vi "avgCoherence.vi"(3 "error in (no error)":errorcluster, 4 "frequency (cycles/period)":dbl, 5 "x2":dbl[](array[numeric]), 6 "x1":dbl[](array[numeric])) -> (0 "error out":errorcluster, 1 "coherence":dbl[](array[numeric]), 2 "coherence at frequency":dbl)   [LabVIEW 2017]
uses:
  <vilib>/measure/maspectr.llb/Frequency Response Function (Mag-Phase) 1-1.vi
  <vilib>/measure/NI_MAPro.lvlib
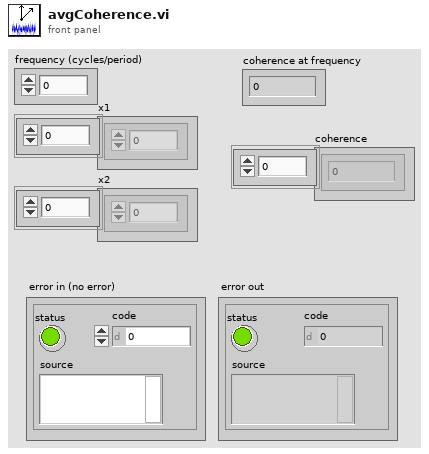
[diagram p1: front panel]
types:
  T1 = cluster{"averaging mode":enum16{"No averaging", "Vector averaging", "RMS averaging", "Peak hold"}, "weighting mode":enum16{"Linear", "Exponential"}, "number of averages":u32}
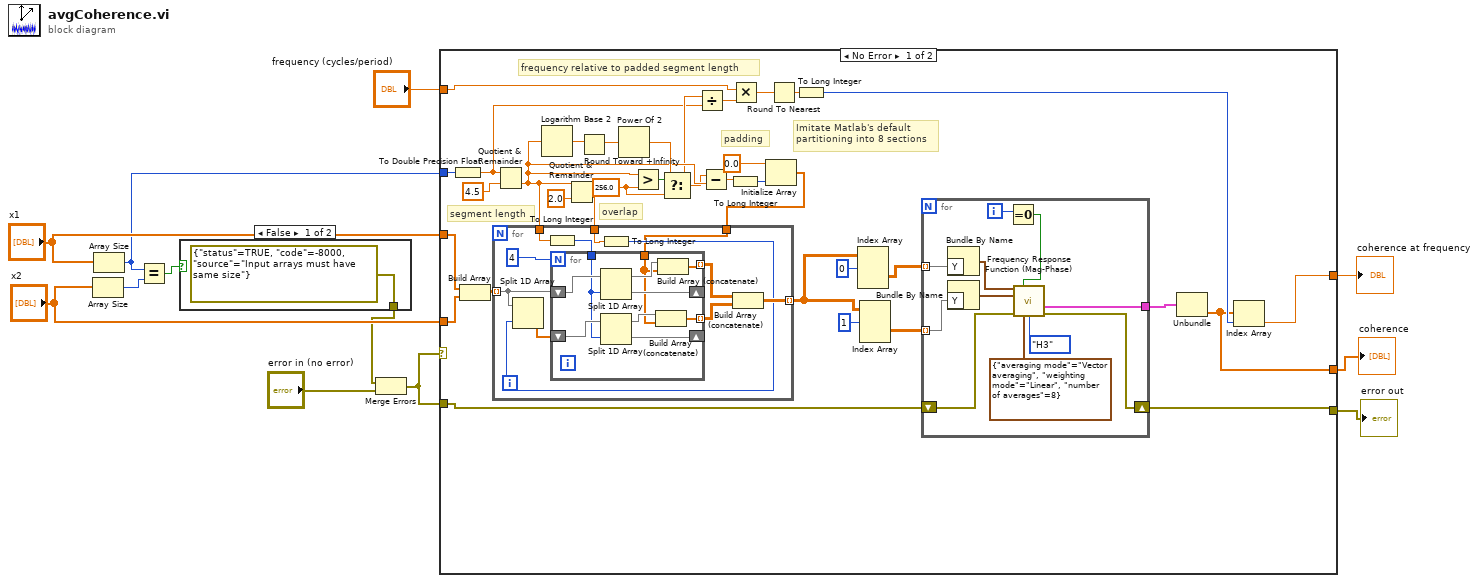
[diagram p0: block diagram]
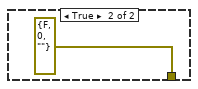
[diagram p2: hidden frame]
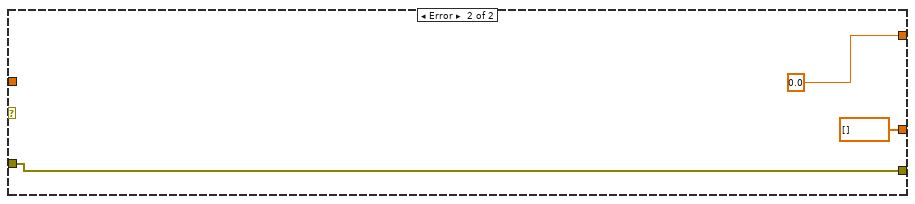
[diagram p3: hidden frame]
diagram:
  n1 = Array Size(array="x2") -> (size(s)=w10:i32)
  n2 = Array Size(array="x1") -> (size(s)=w5:i32)
  n3 = Equal?(x=w5, y=w10) -> (x = y?=w9:bool)
  n4 = case shown="False" w9 {
    tunnel: [errorcluster {"status"=TRUE, "code"=-8000, "source"="Input arrays must have same size"} ("error constant") errorcluster {"status"=FALSE, "code"=0, "source"=""} ("error constant")] -> w8
    frame False {
    }
    frame True {
    }
  }
  n5 = Merge Errors(w8, "error in (no error)") -> (w6:errorcluster)
  n6 = case shown="No Error" w6 {
    tunnel: w6 -> [w48 w83]
    tunnel: "x1" -> [w41 _]
    tunnel: "x2" -> [w40 _]
    tunnel: w5 -> [w46 _]
    tunnel: [w44 w83] -> w4
    tunnel: [w43 0.0 ("Numeric")] -> w3
    tunnel: "frequency (cycles/period)" -> [w22 _]
    tunnel: [w15 dbl[] [] ("coherence")] -> w1
    frame No Error {
      w35 = 256.0 ("y")
      # "frequency relative to padded segment length"
      # "Imitate Matlab's default\npartitioning into 8 sections"
      # "padding"
      # "overlap"
      # "segment length"
      n7 = To Double Precision Float(number=w46) -> (double precision float=w16:dbl)
      n8 = Build Array(w41, w40) -> (w39:dbl[][])
      n9 = Quotient & Remainder(x=w16, y=4.5) -> (floor(x/y)=w18:dbl)  [unwired: 1 out]
      n10 = Logarithm Base 2(1:w18) -> (0:w37:dbl)
      n11 = Quotient & Remainder(x=w18, y=2.0) -> (floor(x/y)=w38:dbl)  [unwired: 1 out]
      n12 = Round Toward +Infinity(x=w37) -> (ceil(x): smallest int >= x=w34:dbl)
      n13 = Power Of 2(x=w34) -> (2^x=w33:dbl)
      n14 = Greater?(x=w18, y=w35) -> (0:w36:bool)
      n15 = Select(t=w33, s=w36, f=w35) -> (s? t:f=w17:dbl)
      n16 = Divide(x=w17, y=w16) -> (x/y=w23:dbl)
      n17 = Subtract(x=w17, y=w18) -> (x-y=w32:dbl)
      n18 = To Long Integer(number=w32) -> (32bit integer=w31:i32)
      n19 = Multiply(x=w22, y=w23) -> (x*y=w20:dbl)
      n20 = Initialize Array(0.0 ("element"), w31) -> (w29:dbl[])
      n21 = for {
        tunnel: w39 -> [w55] mode=indexing
        tunnel: w18 -> [w57]
        tunnel: w38 -> [w54]
        tunnel: [w58] -> w25 mode=indexing
        tunnel: w29 -> [w50]
        n22 = To Long Integer(number=w57) -> (32bit integer=w56:i32)
        n23 = To Long Integer(number=w54) -> (32bit integer=w51:i32)
        n24 = Split 1D Array(array=w55, index=w51) -> (second subarray=w53:dbl[])  [unwired: 1 out]
        n25 = for {
          N: 4 -> [_]
          tunnel: w56 -> [w64]
          shift-right: [w68] -> _
          shift-left: w55 -> [w69]
          shift-right: [w63] -> _
          shift-left: w53 -> [w67]
          tunnel: [w66] -> w52 mode=indexing
          tunnel: w50 -> [w61]
          tunnel: [w60] -> w49 mode=indexing
          n26 = Split 1D Array(array=w69, index=w64) -> (first subarray=w65:dbl[], second subarray=w68:dbl[])
          n27 = Split 1D Array(array=w67, index=w64) -> (first subarray=w62:dbl[], second subarray=w63:dbl[])
          n28 = Build Array (concatenate)(w62, w61) -> (w60:dbl[])
          n29 = Build Array (concatenate)(w65, w61) -> (w66:dbl[])
        }
        n30 = Build Array (concatenate)(w52, w49) -> (w58:dbl[][])
      }
      n31 = Round To Nearest(number=w20) -> (nearest integer value=w21:dbl)
      n32 = To Long Integer(number=w21) -> (32bit integer=w19:i32)
      n33 = Index Array(array=w25, index (dim 0)=0 ("index (page)")) -> (element=w27:dbl[][])  [unwired: 2 in]
      n34 = Index Array(array=w25, index (dim 0)=1 ("index (page)")) -> (element=w24:dbl[][])  [unwired: 2 in]
      n35 = for {
        tunnel: [w78] -> w47
        shift-right: [w74] -> w44
        shift-left: w48 -> [w80]
        tunnel: w27 -> [w71] mode=indexing
        tunnel: w24 -> [w70] mode=indexing
        i -> [w73]
        n36 = Bundle By Name("Y"=w71) -> (w76:waveform(dbl))  [unwired: 1 in]
        n37 = Bundle By Name("Y"=w70) -> (w77:waveform(dbl))  [unwired: 1 in]
        n38 = Equal To 0?(x=w73) -> (x = 0?=w72:bool)
        n39 = call-poly <vilib>:"Frequency Response Function (Mag-Phase).vi"("time signal X"=w76, "restart averaging (F)"=w72, "time signal Y"=w77, "error in (no error)"=w80, "averaging parameters"=T1 {"averaging mode"=enum."Vector averaging", "weighting mode"=enum."Linear", "number of averages"=8}, "FRF Mode"=enum16{"H1", "H2", "H3"}."H3") -> ("coherence"=w78:cluster{"f0":dbl, "df":dbl, "coherence":dbl[]}, "error out"=w74:errorcluster)  [unwired: 4 in, 4 out]
      }
      n40 = Unbundle(w47) -> ("coherence"=w15:dbl[])  [unwired: 2 out]
      n41 = Index Array(array=w15, index=w19) -> (element=w43:dbl)
    }
    frame Error {
    }
  }
  "error out" <- w4
  "coherence at frequency" <- w3
  "coherence" <- w1
